vi "VoltToC.vi"(8 "Offset":dbl, 11 "Thermoelectric Voltage":dbl) -> (3 "Degrees C":dbl)   [LabVIEW 2018]
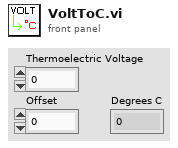
[diagram p1: front panel]
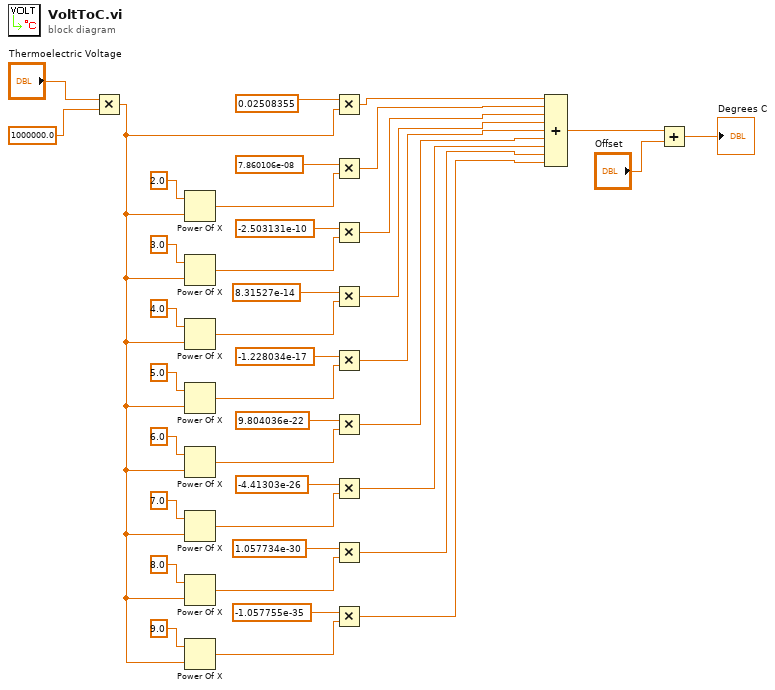
[diagram p0: block diagram]
diagram:
  n1 = Multiply(x="Thermoelectric Voltage", y=1000000.0) -> (x*y=w29:dbl)
  n2 = Power Of X(1:w29, 2:2.0 ("y")) -> (0:w14:dbl)
  n3 = Power Of X(1:w29, 2:3.0 ("y")) -> (0:w16:dbl)
  n4 = Power Of X(1:w29, 2:4.0 ("y")) -> (0:w18:dbl)
  n5 = Power Of X(1:w29, 2:5.0 ("y")) -> (0:w20:dbl)
  n6 = Power Of X(1:w29, 2:6.0 ("y")) -> (0:w22:dbl)
  n7 = Power Of X(1:w29, 2:7.0 ("y")) -> (0:w24:dbl)
  n8 = Power Of X(1:w29, 2:8.0 ("y")) -> (0:w26:dbl)
  n9 = Power Of X(1:w29, 2:9.0 ("y")) -> (0:w28:dbl)
  n10 = Multiply(x=0.02508355, y=w29) -> (x*y=w12:dbl)
  n11 = Multiply(x=7.860106e-08, y=w14) -> (x*y=w11:dbl)
  n12 = Multiply(x=-2.503131e-10, y=w16) -> (x*y=w9:dbl)
  n13 = Multiply(x=8.31527e-14, y=w18) -> (x*y=w8:dbl)
  n14 = Multiply(x=-1.228034e-17, y=w20) -> (x*y=w7:dbl)
  n15 = Multiply(x=9.804036e-22, y=w22) -> (x*y=w6:dbl)
  n16 = Multiply(x=-4.41303e-26, y=w24) -> (x*y=w5:dbl)
  n17 = Multiply(x=1.057734e-30, y=w26) -> (x*y=w4:dbl)
  n18 = Multiply(x=-1.057755e-35, y=w28) -> (x*y=w3:dbl)
  n19 = Compound Arithmetic op=ADD(w12, w11, w9, w8, w7, w6, w5, w4, w3) -> (w10:dbl)
  n20 = Add(x=w10, y="Offset") -> (x+y=→"Degrees C":dbl)
